vi "Arm State Controller (Auto).vi"(0 "Target Arm State":T1(ring)=enum."Intake") -> ()   [LabVIEW 2020]
uses:
  <vilib>/Rock Robotics/WPI/ThirdParty/REV Robotics/REVLib/Typedef/Spark MAX Control Type.ctl
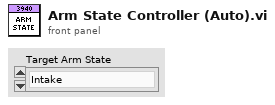
[diagram p1: front panel]
types:
  T1 = enum16{"Manual", "High Cone", "High Cube", "Mid Cone", "Mid Cube", "Intake", "Cube Handoff", "Cone Handoff", "Stow"}
  T2 = typedef "Spark MAX Control Type.ctl" = enum16{"Percent VBus", "Voltage", "Velocity", "Position", "Smart Motion", "Current", "Smart Velocity"}
  T3 = cluster{"Stow Shoulder Setpoint":dbl, "Intake Shoulder Setpoint":dbl, "Cube Handoff Shoulder Setpoint":dbl, "Cone Handoff Shoulder Setpoint":dbl, "Mid Cone Shoulder Setpoint":dbl, "Mid Cube Shoulder Setpoint":dbl, "High Cone Shoulder Setpoint":dbl, "High Cube Shoulder Setpoint":dbl}
  T4 = cluster{"Stow Elbow Setpoint":dbl, "Intake Elbow Setpoint":dbl, "Cube Handoff Elbow Setpoint":dbl, "Cone Handoff Elbow Setpoint":dbl, "Mid Cone Elbow Setpoint":dbl, "Mid Cube Elbow Setpoint":dbl, "High Cone Elbow Setpoint":dbl, "High Cube Elbow Setpoint":dbl}
  T5 = typedef "WPI_MotorControlDeviceRef.ctl" = cluster{"DeviceStatus":errorcluster, "Type":T6, "PWM":cluster{"PWM Channel":T7, "DeadBand":T8}, "CAN":cluster{"Device Number":u8, "SetOutput VI Ref":variant, "GetOutput VI Ref":variant, "Enable VI Ref":variant, "Disable VI Ref":variant, "Data":variant}, "Invert":bool, "DIO PWM":cluster{"PWM \"Enable\" Channel":T7, "DIOChannel":T9, "PWM Rate":dbl}}
  T6 = typedef "WPI_MotorControlType.ctl" = enum16{"PWM", "CAN", "DIO PWM"}
  T7 = typedef "FPGA_DIOPWMChannel.ctl" = enum8{"PWM 0", "PWM 1", "PWM 2", "PWM 3", "PWM 4", "PWM 5", "PWM 6", "PWM 7", "PWM 8", "PWM 9", "PWM MXP 0", "PWM MXP 1", "PWM MXP 2", "PWM MXP 3", "PWM MXP 4", "PWM MXP 5", "PWM MXP 6", "PWM MXP 7", "PWM MXP 8", "PWM MXP 9", "Invalid"}
  T8 = typedef "WPI_PWMDeadband.ctl" = cluster{"Name":string, "maxPositivePwm":i32, "minPositivePwm":i32, "centerPwm":i32, "maxNegativePwm":i32, "minNegativePwm":i32, "angularRange":u16}
  T9 = typedef "FPGA_DIOChannel.ctl" = enum8{"DIO 0", "DIO 1", "DIO 2", "DIO 3", "DIO 4", "DIO 5", "DIO 6", "DIO 7", "DIO 8", "DIO 9", "DIO MXP 0", "DIO MXP 1", "DIO MXP 2", "DIO MXP 3", "DIO MXP 4", "DIO MXP 5", "DIO MXP 6", "DIO MXP 7", "DIO MXP 8", "DIO MXP 9", "DIO MXP 10", "DIO MXP 11", "DIO MXP 12", "DIO MXP 13", "DIO MXP 14", "DIO MXP 15", "SPI Port CS1", "SPI Port CS2", "SPI Port CS3", "SPI Port MISO", "SPI Port MOSI", "Invalid"}
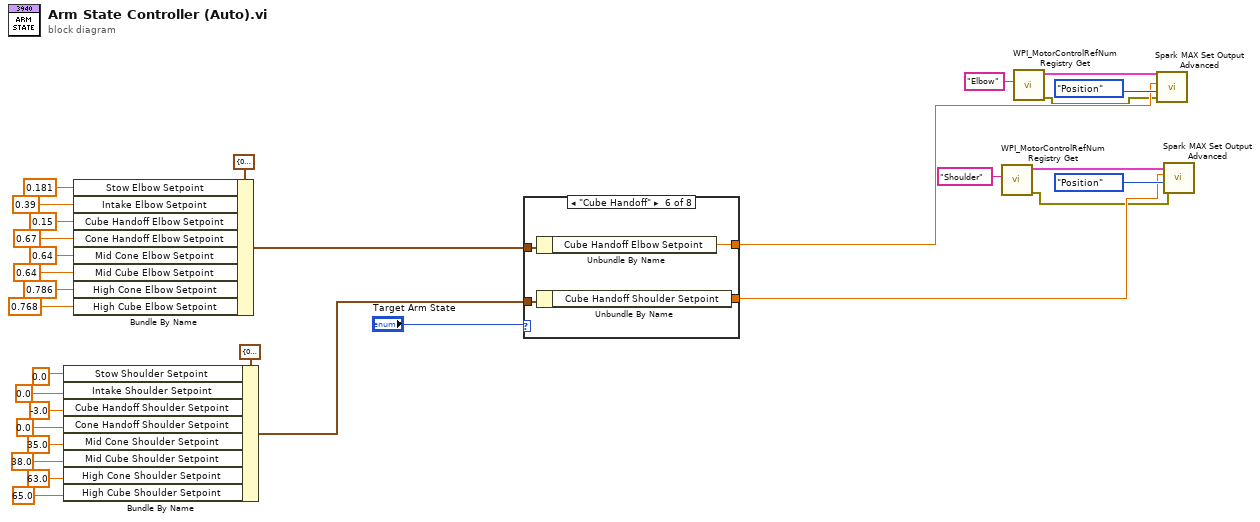
[diagram p0: block diagram]
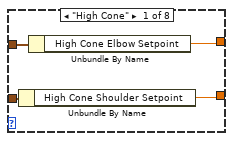
[diagram p2: hidden frame]
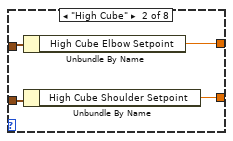
[diagram p3: hidden frame]
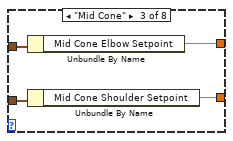
[diagram p4: hidden frame]
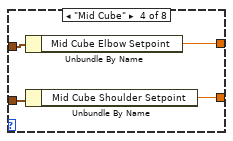
[diagram p5: hidden frame]
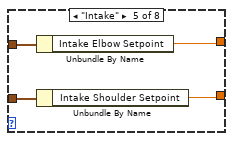
[diagram p6: hidden frame]
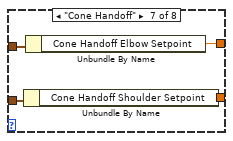
[diagram p7: hidden frame]
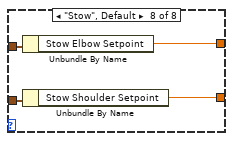
[diagram p8: hidden frame]
diagram:
  n1 = Bundle By Name(cluster=T3 {"Stow Shoulder Setpoint"=0.0, "Intake Shoulder Setpoint"=0.0, "Cube Handoff Shoulder Setpoint"=0.0, "Cone Handoff Shoulder Setpoint"=0.0, "Mid Cone Shoulder Setpoint"=0.0, "Mid Cube Shoulder Setpoint"=0.0, "High Cone Shoulder Setpoint"=0.0, "High Cube Shoulder Setpoint"=0.0}, "Stow Shoulder Setpoint"=0.0 ("Stow Elbow Setpoint"), "Intake Shoulder Setpoint"=0.0 ("Intake Elbow Setpoint"), "Cube Handoff Shoulder Setpoint"=-3.0 ("Cube Handoff Elbow Setpoint"), "Cone Handoff Shoulder Setpoint"=0.0 ("Cone Handoff Elbow Setpoint"), "Mid Cone Shoulder Setpoint"=35.0 ("Mid Cone Elbow Setpoint"), "Mid Cube Shoulder Setpoint"=38.0 ("Mid Cube Elbow Setpoint"), "High Cone Shoulder Setpoint"=63.0 ("High Cone Elbow Setpoint"), "High Cube Shoulder Setpoint"=65.0 ("High Cube Elbow Setpoint")) -> (w26:T3)
  n2 = Bundle By Name(cluster=T4 {"Stow Elbow Setpoint"=0.0, "Intake Elbow Setpoint"=0.0, "Cube Handoff Elbow Setpoint"=0.0, "Cone Handoff Elbow Setpoint"=0.0, "Mid Cone Elbow Setpoint"=0.0, "Mid Cube Elbow Setpoint"=0.0, "High Cone Elbow Setpoint"=0.0, "High Cube Elbow Setpoint"=0.0}, "Stow Elbow Setpoint"=0.181, "Intake Elbow Setpoint"=0.39, "Cube Handoff Elbow Setpoint"=0.15, "Cone Handoff Elbow Setpoint"=0.67, "Mid Cone Elbow Setpoint"=0.64, "Mid Cube Elbow Setpoint"=0.64, "High Cone Elbow Setpoint"=0.786, "High Cube Elbow Setpoint"=0.768) -> (w27:T4)
  n3 = case shown="\"Cube Handoff\"" "Target Arm State" {
    tunnel: [w35 w39 w43 w47 w51 w55 w59 w63] -> w20
    tunnel: [w34 w38 w42 w46 w50 w54 w58 w62] -> w22
    tunnel: w27 -> [w33 w37 w41 w45 w49 w53 w57 w61]
    tunnel: w26 -> [w32 w36 w40 w44 w48 w52 w56 w60]
    frame "High Cone" {
      n4 = Unbundle By Name(w32) -> ("High Cone Shoulder Setpoint"=w34:dbl)
      n5 = Unbundle By Name(w33) -> ("High Cone Elbow Setpoint"=w35:dbl)
    }
    frame "High Cube" {
      n6 = Unbundle By Name(w37) -> ("High Cube Elbow Setpoint"=w39:dbl)
      n7 = Unbundle By Name(w36) -> ("High Cube Shoulder Setpoint"=w38:dbl)
    }
    frame "Mid Cone" {
      n8 = Unbundle By Name(w41) -> ("Mid Cone Elbow Setpoint"=w43:dbl)
      n9 = Unbundle By Name(w40) -> ("Mid Cone Shoulder Setpoint"=w42:dbl)
    }
    frame "Mid Cube" {
      n10 = Unbundle By Name(w45) -> ("Mid Cube Elbow Setpoint"=w47:dbl)
      n11 = Unbundle By Name(w44) -> ("Mid Cube Shoulder Setpoint"=w46:dbl)
    }
    frame "Intake" {
      n12 = Unbundle By Name(w49) -> ("Intake Elbow Setpoint"=w51:dbl)
      n13 = Unbundle By Name(w48) -> ("Intake Shoulder Setpoint"=w50:dbl)
    }
    frame "Cube Handoff" {
      n14 = Unbundle By Name(w53) -> ("Cube Handoff Elbow Setpoint"=w55:dbl)
      n15 = Unbundle By Name(w52) -> ("Cube Handoff Shoulder Setpoint"=w54:dbl)
    }
    frame "Cone Handoff" {
      n16 = Unbundle By Name(w56) -> ("Cone Handoff Shoulder Setpoint"=w58:dbl)
      n17 = Unbundle By Name(w57) -> ("Cone Handoff Elbow Setpoint"=w59:dbl)
    }
    frame "Stow", Default {
      n18 = Unbundle By Name(w61) -> ("Stow Elbow Setpoint"=w63:dbl)
      n19 = Unbundle By Name(w60) -> ("Stow Shoulder Setpoint"=w62:dbl)
    }
  }
  n20 = call <vilib>:"WPI_MotorControlRefNum Registry Get.vi"("refnum name"="Shoulder") -> ("error out"=w17:errorcluster, "MotorControlDevRef"=w21:T5)  [unwired: 9 in]
  n21 = call <vilib>:"WPI_MotorControlRefNum Registry Get.vi"("refnum name"="Elbow") -> ("error out"=w18:errorcluster, "MotorControlDevRef"=w24:T5)  [unwired: 9 in]
  n22 = call <vilib>:"Spark MAX Set Output Advanced.vi"("error in (no error)"=w18, "Control Mode"=Spark_MAX_Control_Type."Position", "Setpoint"=w20, "MotorControlDevRef"=w24) -> ()  [unwired: 6 in, 2 out]
  n23 = call <vilib>:"Spark MAX Set Output Advanced.vi"("error in (no error)"=w17, "Control Mode"=Spark_MAX_Control_Type."Position", "Setpoint"=w22, "MotorControlDevRef"=w21) -> ()  [unwired: 6 in, 2 out]
